vi "Update Project Config.vi"(8 "error in (no error)":errorcluster, 10 "Array":refnum<vi>[](array[refnum]), 11 "Refnum in":T1) -> (0 "error out":errorcluster)   [LabVIEW 2018]
uses:
  <vilib>/addons/database/Connection.llb/Conn ObjectReference.ctl
  <vilib>/addons/database/Connection.llb/Conn Execute.vi
  <vilib>/addons/database/NI_Database_API.lvlib
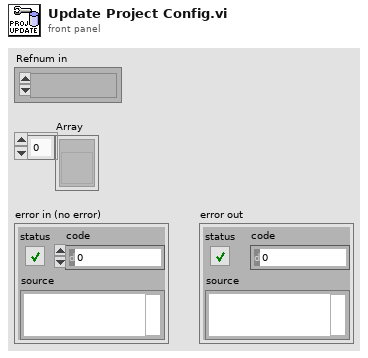
[diagram p1: front panel]
types:
  T1 = typedef "NI_Database_API.lvlib/Conn ObjectReference.ctl" = refnum<k1>
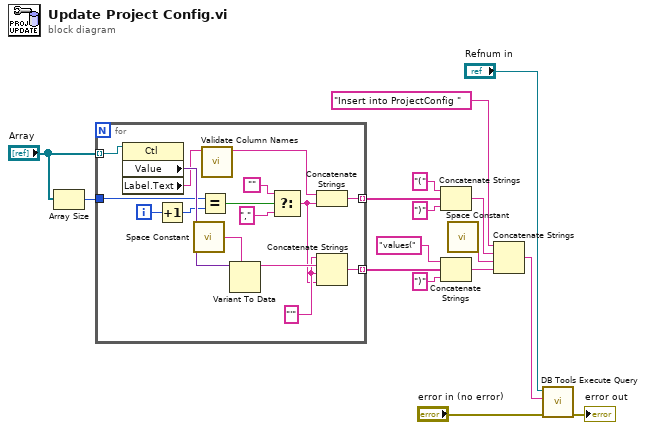
[diagram p0: block diagram]
diagram:
  n1 = Array Size(array="Array") -> (size(s)=w16:i32)
  n2 = for {
    tunnel: "Array" -> [w32] mode=indexing
    tunnel: [w25] -> w9 mode=indexing
    tunnel: [w26] -> w8 mode=indexing
    tunnel: w16 -> [w23]
    i -> [w22]
    w24 = "'" ("string")
    n3 = property class="Ctl"(reference=w32) -> ("Value"=w31:variant, "Label.Text"=w29:string)  [unwired: 1 in, 2 out]
    n4 = Increment(x=w22) -> (x+1=w21:i32)
    n5 = call <vilib>:"Space Constant.vi"() -> ("String"=w30:string)
    n6 = Equal?(x=w23, y=w21) -> (x = y?=w20:bool)
    n7 = call "Validate Column Names.vi"("Label.Text"=w29) -> ("result string"=w28:string)  [unwired: 9 in, 1 out]
    n8 = Variant To Data(type=w30, Variant=w31) -> (data=w27:string)  [unwired: 1 in, 1 out]
    n9 = Select(t="", s=w20, f="," ("string")) -> (s? t:f=w18:string)
    n10 = Concatenate Strings(w28, w18) -> (w26:string)
    n11 = Concatenate Strings(w24, w27, w24, w18) -> (w25:string)
  }
  n12 = Concatenate Strings("(" ("string"), w8, ")") -> (w12:string)
  n13 = Concatenate Strings("values(" ("string"), w9, ")" ("string")) -> (w13:string)
  n14 = call <vilib>:"Space Constant.vi"() -> ("String"=w11:string)
  n15 = Concatenate Strings("Insert into ProjectConfig ", w12, w11, w13) -> (w14:string)
  n16 = call-poly <vilib>:"DB Tools Execute Query.vi"("error in (no error)"="error in (no error)", "SQL query"=w14, "connection reference"="Refnum in") -> ("error out"=→"error out":errorcluster)  [unwired: 5 in, 1 out]
